vi "_Recursively Set Fp Cluster Autosizing Property.vi"(8 "error in (no error)":errorcluster, 10 "type":T1(ring), 11 "SelList[]":refnum<vi>[](array[refnum])) -> (0 "error out":errorcluster, 3 "Changed":bool)   [LabVIEW 2012, in "Cluster AutoSizing.lvlib"]
uses:
  Cluster AutoSizing.lvlib
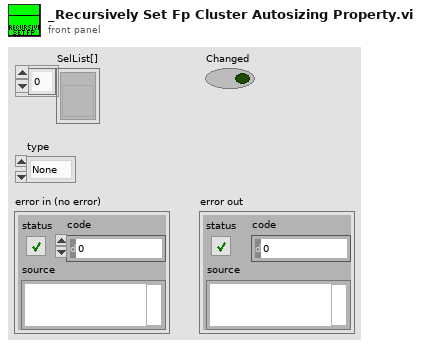
[diagram p1: front panel]
types:
  T1 = enum16{"None", "Size to Fit", "Arrange Horizontally", "Arrange Veritcally"}
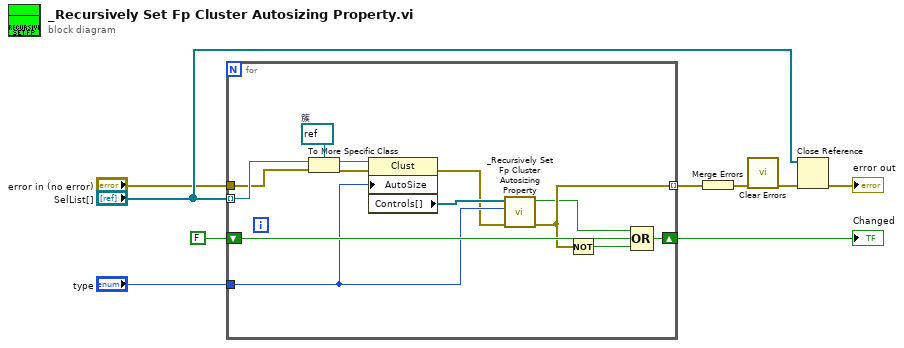
[diagram p0: block diagram]
diagram:
  n1 = for {
    shift-right: [w21] -> w3
    shift-left: FALSE -> [w22]
    tunnel: "SelList[]" -> [w20] mode=indexing
    tunnel: "error in (no error)" -> [w17]
    tunnel: [w11] -> w4 mode=indexing
    tunnel: "type" -> [w13]
    w18 = refnum<vi> refnum  # 簇
    n2 = To More Specific Class(target class=w18, reference=w20, error in=w17) -> (specific class reference=w19:refnum<vi>, error out=w16:errorcluster)
    n3 = property class="Clust"(reference=w19, error in=w16, "AutoSize"=w13) -> (error out=w12:errorcluster, "Controls[]"=w14:refnum<vi>[])  [unwired: 1 out]
    n4 = call "_Recursively Set Fp Cluster Autosizing Property.vi"("error in (no error)"=w12, "type"=w13, "SelList[]"=w14) -> ("error out"=w11:errorcluster, "Changed"=w10:bool)  [unwired: 7 in]
    n5 = Not(x=w11) -> (.not. x?=w15:bool)
    n6 = Compound Arithmetic op=OR(w10, w22, w15) -> (w21:bool)
  }
  "Changed" <- w3
  n7 = Merge Errors(w4) -> (w6:errorcluster)
  n8 = call <vilib>:"Clear Errors.vi"("error in (no error)"=w6) -> ("error out"=w7:errorcluster)  [unwired: 6 in]
  n9 = Close Reference(reference="SelList[]", error in (no error)=w7) -> (error out=→"error out":errorcluster)
